vi "Helm State Machine Cycle.vi"(8 "error in (no error)":errorcluster, 11 "RDS Helm Actor in":refnum<class "RDS Helm Actor.lvclass">) -> (0 "error out":errorcluster, 3 "RDS Helm Actor out":refnum<class "RDS Helm Actor.lvclass">)   [LabVIEW 2015, in "RDS Helm Actor.lvlib" / "RDS Helm Actor.lvclass"]
uses:
  RDS Helm Actor.lvclass
  RDS Helm Actor.lvclass/RDS Helm Actor.ctl
  Libraries/RDS Child Messages/Helm/Steering Command/Steering Command Cntrl.ctl
  Libraries/RDS Child Messages/Helm/Heading Command/Heading Command Cntrl.ctl
  Libraries/RDS Child Messages/RDS Child Messages.lvlib
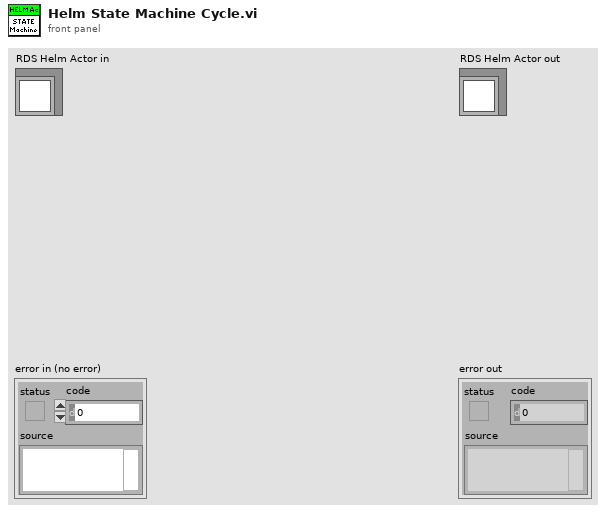
[diagram p1: front panel]
types:
  T1 = typedef "RDS Child Messages.lvlib/Heading Command Cntrl.ctl" = cluster{"Throttle":i16, "Heading":sgl, "Duration (s)":i16}
  T2 = typedef "RDS Child Messages.lvlib/Steering Command Cntrl.ctl" = cluster{"Throttle":i16, "Rudder":i8, "Duration (s)":u16}
  T3 = typedef "RDS Helm Actor.lvlib/Helm State.ctl" = enum16{"Idle", "Executing Heading Command", "Executing Steering Command"}
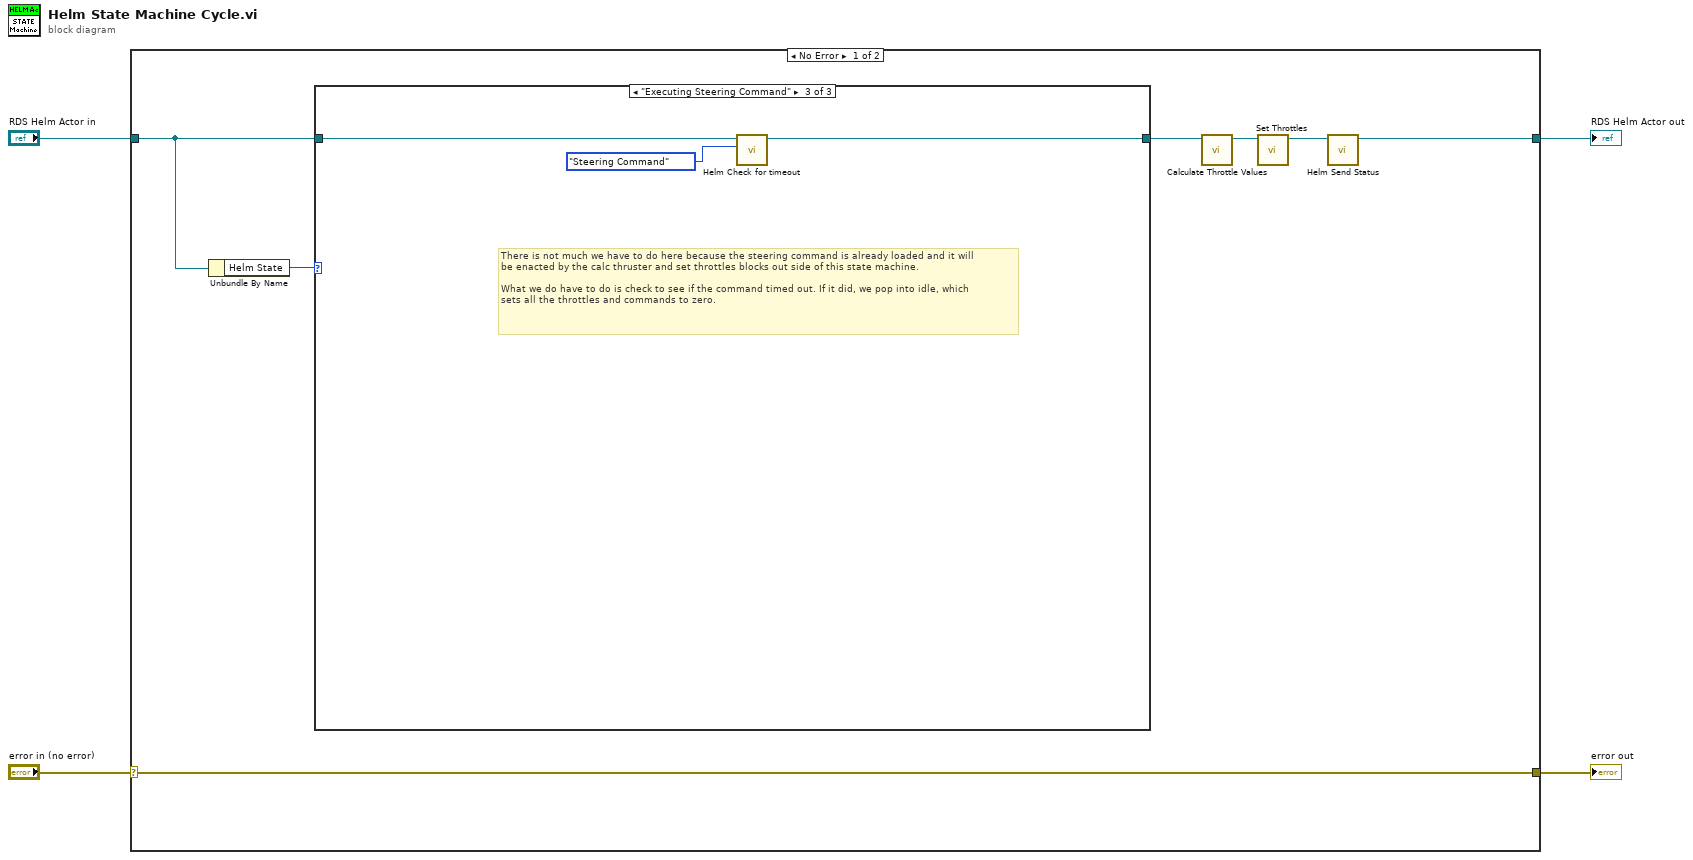
[diagram p0: block diagram]
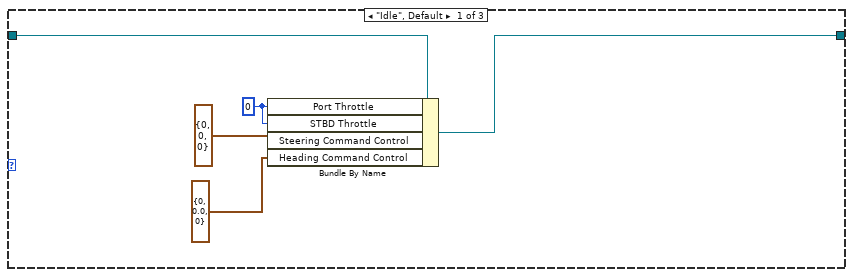
[diagram p2: hidden frame]
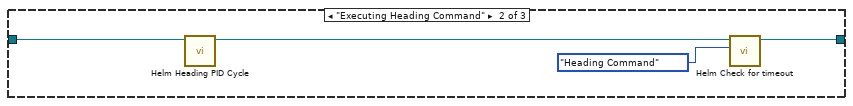
[diagram p3: hidden frame]
diagram:
  n1 = case shown="No Error" "error in (no error)" {
    selector: "error in (no error)" -> [w11 w25]
    tunnel: [w11 w25] -> w3
    tunnel: [w5 w24] -> w1
    tunnel: "RDS Helm Actor in" -> [w10 w24]
    frame No Error {
      n2 = Unbundle By Name(w10) -> ("Helm State"=w9:T3)
      n3 = case shown="\"Executing Steering Command\"" w9 {
        tunnel: [w14 w19 w22] -> w8
        tunnel: w10 -> [w15 w18 w23]
        frame "Idle", Default {
          w16 = i16 0 ("Port Throttle")
          n4 = Bundle By Name(cluster=w15, "Port Throttle"=w16, "STBD Throttle"=w16, "Steering Command Control"=T2 {"Throttle"=0, "Rudder"=0, "Duration (s)"=0}, "Heading Command Control"=T1 {"Throttle"=0, "Heading"=0.0, "Duration (s)"=0}) -> (w14:refnum<class "RDS Helm Actor.lvclass">)
        }
        frame "Executing Heading Command" {
          n5 = call "Helm Heading PID Cycle.vi"("RDS Helm Actor in"=w18) -> ("RDS Helm Actor out"=w17:refnum<class "RDS Helm Actor.lvclass">)  [unwired: 9 in, 1 out]
          n6 = call "Helm Check for timeout.vi"("Command"=enum16{"Steering Command", "Heading Command"}."Heading Command", "RDS Helm Actor in"=w17) -> ("RDS Helm Actor out"=w19:refnum<class "RDS Helm Actor.lvclass">)  [unwired: 8 in, 1 out]
        }
        frame "Executing Steering Command" {
          # "There is not much we have to do here because the steering command is already loaded and it will\nbe enacted by the calc thruster and set throttles blocks out side of this state machine. \n\nWhat we do have to do is check to see if the command timed out. If it did, we pop into idle, which\nsets all the throttles and commands to zero."
          n7 = call "Helm Check for timeout.vi"("Command"=enum16{"Steering Command", "Heading Command"}."Steering Command", "RDS Helm Actor in"=w23) -> ("RDS Helm Actor out"=w22:refnum<class "RDS Helm Actor.lvclass">)  [unwired: 8 in, 1 out]
        }
      }
      n8 = call "Calculate Throttle Values.vi"("RDS Helm Actor in"=w8) -> ("RDS Helm Actor out"=w7:refnum<class "RDS Helm Actor.lvclass">)  [unwired: 9 in, 1 out]
      n9 = call "Set Throttles.vi"("RDS Helm Actor in"=w7) -> ("RDS Helm Actor out"=w6:refnum<class "RDS Helm Actor.lvclass">)  [unwired: 9 in, 1 out]
      n10 = call "Helm Send Status.vi"("RDS Helm Actor in"=w6) -> ("RDS Helm Actor out"=w5:refnum<class "RDS Helm Actor.lvclass">)  [unwired: 9 in, 1 out]
    }
    frame Error {
    }
  }
  "error out" <- w3
  "RDS Helm Actor out" <- w1
